vi "Add Library To Project.vi"(8 "error in":errorcluster, 11 "First Library Script Strategy in":refnum<class "First Library Script Strategy.lvclass">) -> (0 "error out":errorcluster)   [LabVIEW 2021, in "_Create From Template.lvlib" / "Script Strategy.lvlib" / "First Library Script Strategy.lvclass"]
uses:
  First Library Script Strategy.lvclass
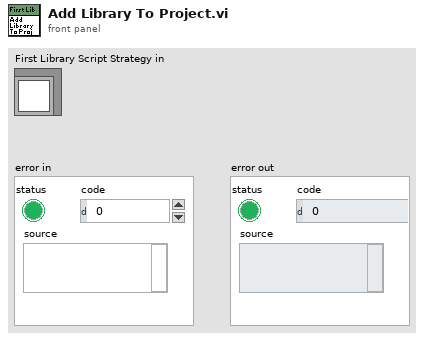
[diagram p1: front panel]
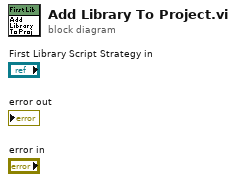
[diagram p0: block diagram]
diagram:
